vi "InstrumentControl.vi"(1 "Close VISA?":bool, 3 "Position":refnum<vi>, 5 "Status":refnum<vi>, 6 "Home fail":refnum<vi>, 7 "Busy":refnum<vi>, 8 "error":errorcluster, 9 "Open VISA?":bool, 10 "Input Message":string, 11 "HomeDone":refnum<vi>) -> (0 "error out":errorcluster, 2 "Output Message":string)   [LabVIEW 2018]
uses:
  QuickSilver/QuickSilver.lvclass
  D:/AOPD/TCSPD/Versoes TCSPD/21 - 160 - TCSPD_TRABALHO_BACKUP 2025-05-19/TCSPD_TRABALHO/Coude/Device/Device.lvclass
  Controlador/Motor/Motor.lvclass
  Controlador/Rele/Rele.lvclass
  Device/Device.lvclass
  Controlador/Comm/COMM.lvclass
  <vilib>/Utility/error.llb/DialogType.ctl
panel:
  in  "UART1":refnum<class "COMM.lvclass">
  in  "Device.lvclass":refnum<class "Device.lvclass">
  in  "LAMPADA":refnum<class "Rele.lvclass">
  in  "REDE":refnum<class "Motor.lvclass">
  in  "ESPELHO":refnum<class "QuickSilver.lvclass">
  in  "PRISMA":refnum<class "QuickSilver.lvclass">
  in  "FENDA":refnum<class "QuickSilver.lvclass">
  out "PAR":string
  out "CMD":string
  out "MEC":string
  # "Objects from Device -> Controlador class"
  # "Objects from Device -> QuickSilver class"
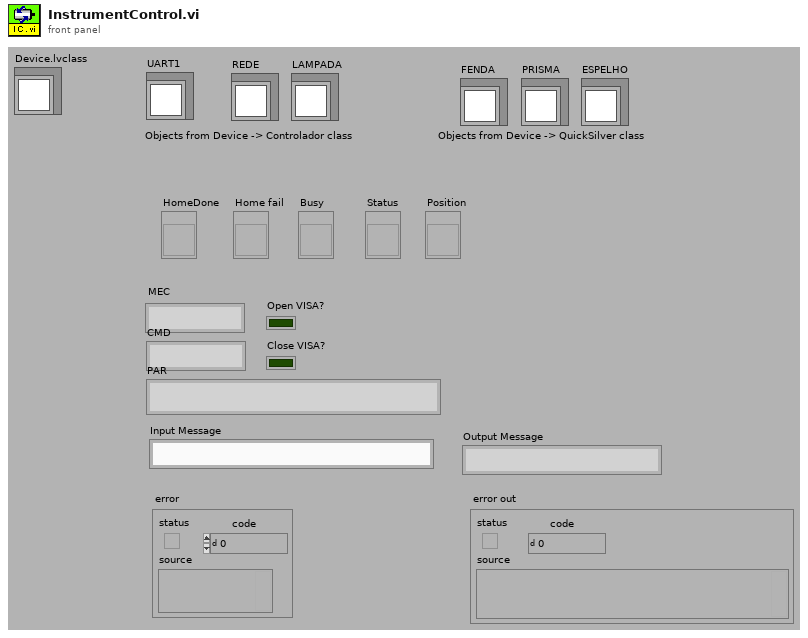
[diagram p1: front panel]
types:
  T1 = typedef "DialogType.ctl" = u16
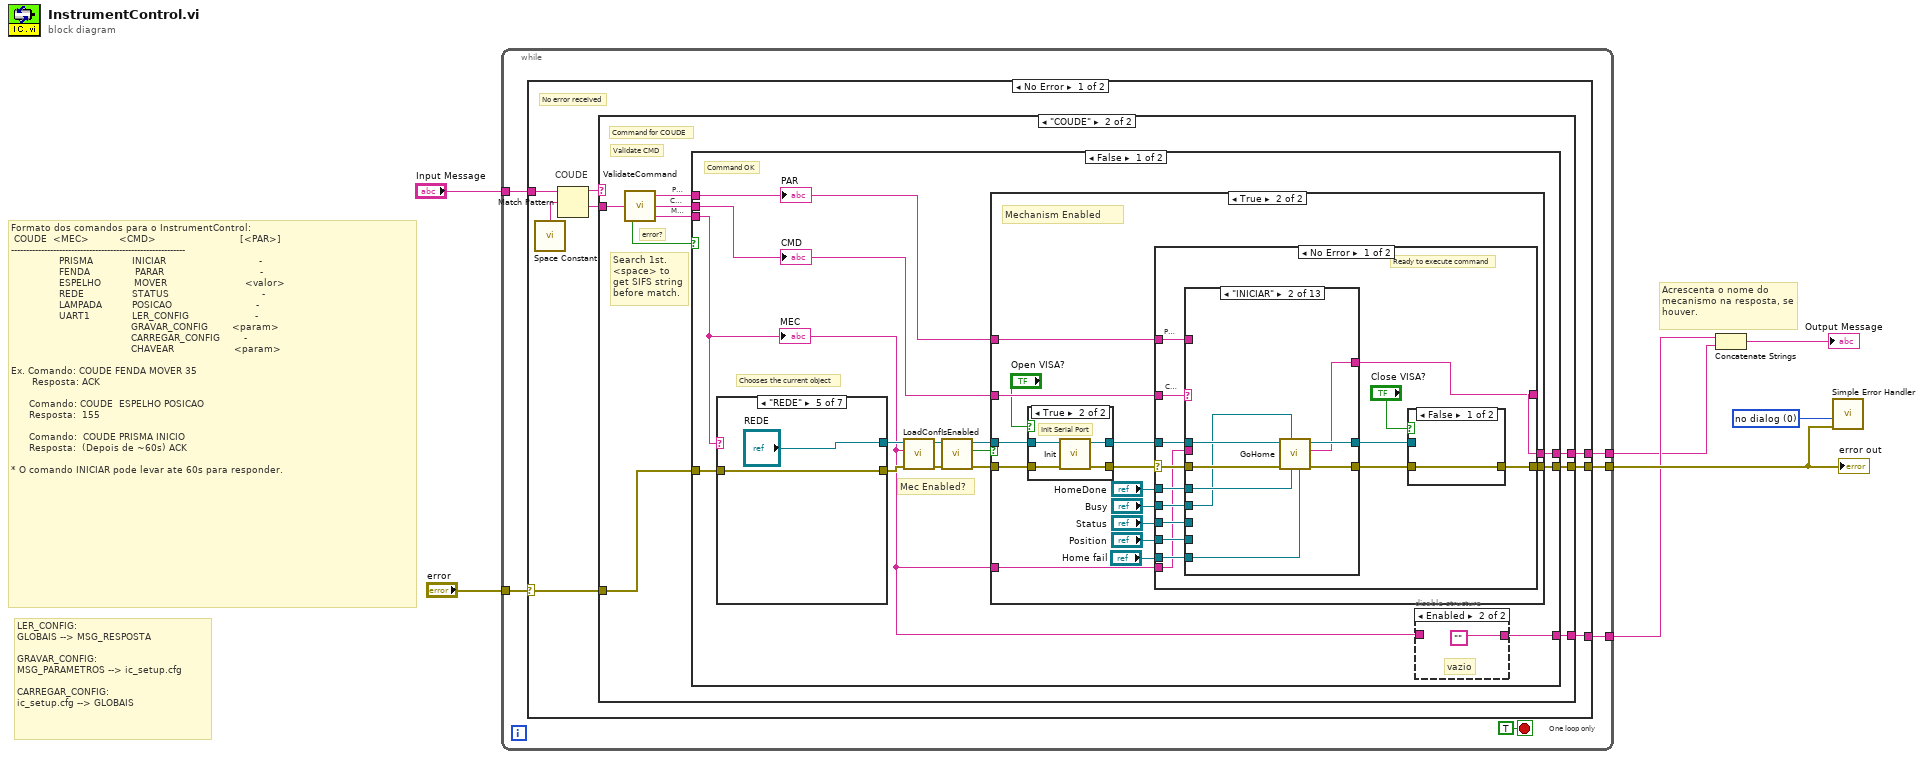
[diagram p0: block diagram]
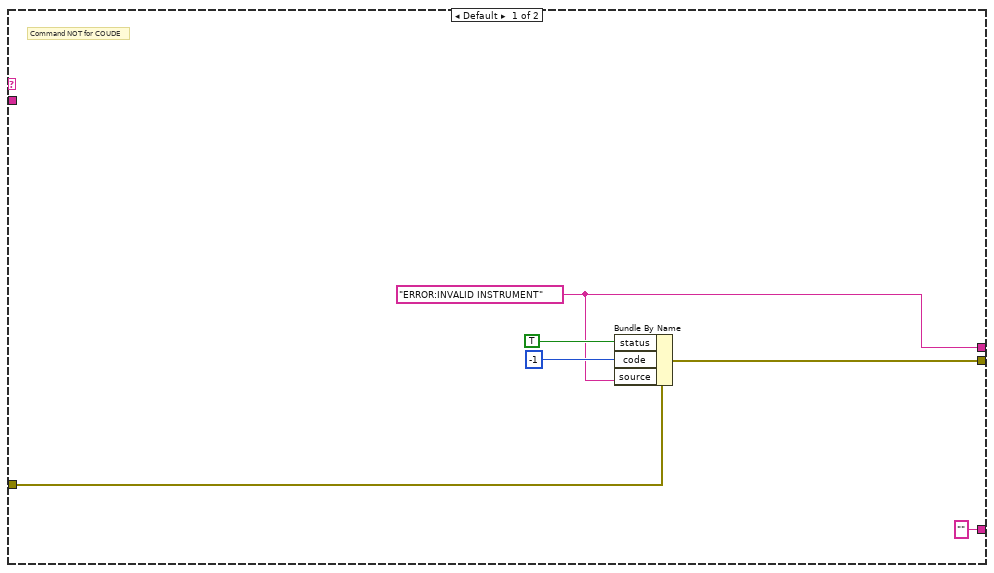
[diagram p2: hidden frame]
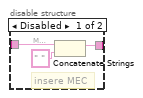
[diagram p3: hidden frame]
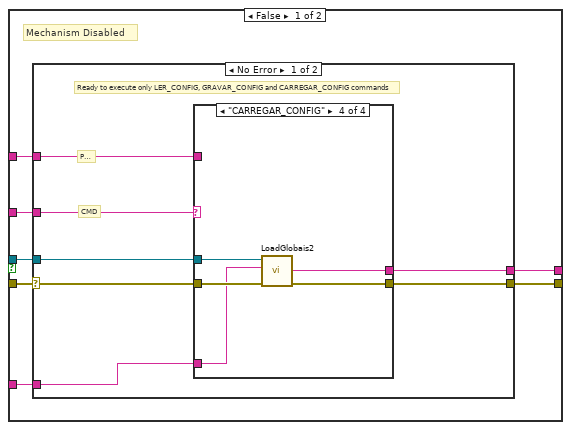
[diagram p4: hidden frame]
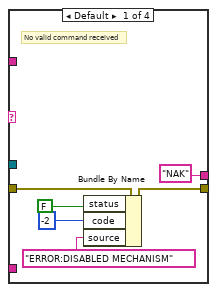
[diagram p5: hidden frame]
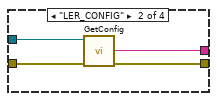
[diagram p6: hidden frame]
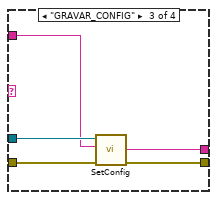
[diagram p7: hidden frame]
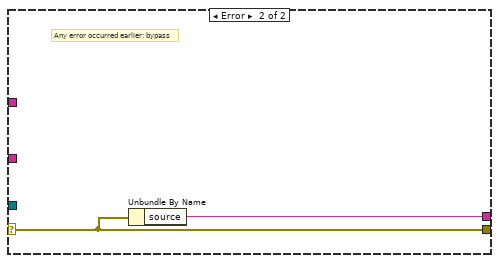
[diagram p8: hidden frame]
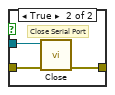
[diagram p10: hidden frame]
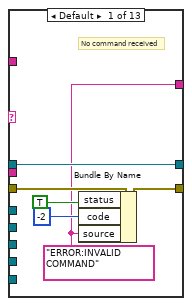
[diagram p11: hidden frame]
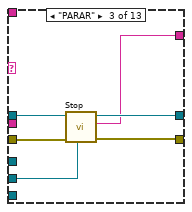
[diagram p12: hidden frame]
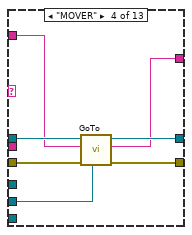
[diagram p13: hidden frame]
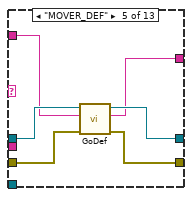
[diagram p14: hidden frame]
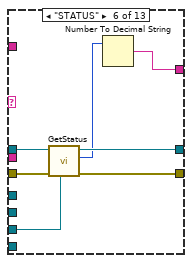
[diagram p15: hidden frame]
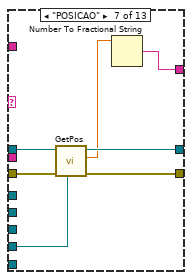
[diagram p16: hidden frame]
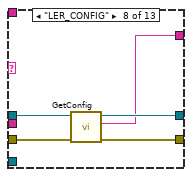
[diagram p17: hidden frame]
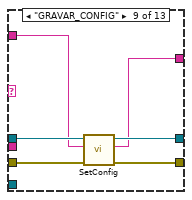
[diagram p18: hidden frame]
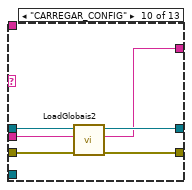
[diagram p19: hidden frame]
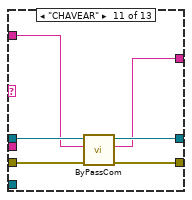
[diagram p20: hidden frame]
diagram:
  w7 = T1 0 items=["no dialog", "OK message", "continue or stop message", "OK message + warnings", "continue/stop + warnings"] ("type of dialog (OK msg:1)")
  # "LER_CONFIG:\nGLOBAIS --> MSG_RESPOSTA\n\nGRAVAR_CONFIG:\nMSG_PARAMETROS --> ic_setup.cfg\n\nCARREGAR_CONFIG:\nic_setup.cfg --> GLOBAIS"
  # "Acrescenta o nome do mecanismo na resposta, se houver."
  # "Formato dos comandos para o InstrumentControl:\n COUDE  <MEC>          <CMD>                            [<PAR>]\n----------------------------------------------------------\n                PRISMA             INICIAR                               -\n                FENDA               PARAR                                -  \n                ESPELHO           MOVER                          <valor>                 \n                REDE                STATUS                               -\n                LAMPADA          POSICAO                            -\n                UART1              LER_CONFIG                      -\n                                        GRAVAR_CONFIG        <param>\n                                        CARREGAR_CONFIG        -\n                                        CHAVEAR                    <param>\n          \nEx. Comando: COUDE FENDA MOVER 35\n       Resposta: ACK\n    \n      Comando: COUDE  ESPELHO POSICAO\n      Resposta:  155\n\n      Comando:  COUDE PRISMA INICIO\n      Resposta:  (Depois de ~60s) ACK \n\n* O comando INICIAR pode levar ate 60s para responder."
  n1 = while {
    tunnel: [w10] -> w6
    tunnel: "Input Message" -> [w12]
    tunnel: "error" -> [w11]
    tunnel: [w9] -> w3
    tunnel: [w8] -> w1
    stop <- TRUE ("stop") stop-if-true
    # "One loop only"
    n2 = case shown="No Error" w11 {
      selector: w11 -> [w21 w239]
      tunnel: [w17 w239] -> w10
      tunnel: w12 -> [w16 _]
      tunnel: [w15 ""] -> w9
      tunnel: [w14 "NAK"] -> w8
      frame No Error {
        # "No error received"
        # "COUDE"
        n3 = call <vilib>:"Space Constant.vi"() -> ("String"=w20:string)
        n4 = Match Pattern(string=w16, regular expression=w20) -> (before substring=w18:string, after substring=w19:string)  [unwired: 3 out]
        n5 = case shown="\"COUDE\"" w18 {
          tunnel: w19 -> [_ w36]
          tunnel: w21 -> [w24 w31]
          tunnel: [w25 w30] -> w17
          tunnel: ["" w29] -> w15
          tunnel: [w22 w28] -> w14
          frame Default {
            w22 = "ERROR:INVALID INSTRUMENT" ("source")
            # "Command NOT for COUDE"
            n6 = Bundle By Name(cluster=w24, "status"=TRUE, "code"=-1, "source"=w22) -> (w25:errorcluster)
          }
          frame "COUDE" {
            # "Search 1st.\n<space> to\nget SIFS string\nbefore match."
            # "MEC"
            # "CMD"
            # "PAR"
            # "Command for COUDE"
            # "Validate CMD"
            # "error?"
            n7 = call "ValidateCommand.vi"("input message 4"=w36) -> ("MECH"=w32:string, "CMD"=w33:string, "PARAM"=w34:string, "err_out"=w35:bool)  [unwired: 1 out]
            n8 = case shown="False" w35 {
              tunnel: w34 -> [w50 _]
              tunnel: w33 -> [w49 _]
              tunnel: w32 -> [w37 _]
              tunnel: w31 -> [w48 w236]
              tunnel: [w45 w235] -> w30
              tunnel: [w39 ""] -> w29
              tunnel: [w38 w231] -> w28
              frame False {
                # "Mec Enabled?"
                # "Chooses the current object"
                # "Command OK"
                n9 = case shown="\"REDE\"" w37 {
                  tunnel: w48 -> [w215 w220 w221 w223 w226 w227 w230]
                  tunnel: [w214 w220 w221 w223 w226 w227 w230] -> w46
                  tunnel: ["Device.lvclass" "FENDA" "PRISMA" "ESPELHO" "REDE" "LAMPADA" "UART1"] -> w47
                  frame Default {
                    # "No valid mechanism received"
                    n10 = Bundle By Name(cluster=w215, "status"=TRUE, "code"=-1, "source"="NAK : INVALID MECHANISM") -> (w214:errorcluster)
                  }
                  frame "FENDA" {
                  }
                  frame "PRISMA" {
                  }
                  frame "ESPELHO" {
                  }
                  frame "REDE" {
                  }
                  frame "LAMPADA" {
                  }
                  frame "SERIAL" {
                  }
                }
                n11 = call-dynamic "LoadConf.vi"("error in"=w46, "MEC"=w37, "Device in"=w47) -> ("error out"=w43:errorcluster, "Device out"=w44:refnum<class "Device.lvclass">)  [unwired: 7 out]
                n12 = call-dynamic "IsEnabled.vi"("error in (no error)"=w43, "Device in"=w44) -> ("error out"=w40:errorcluster, "Boolean"=w42:bool, "Device out"=w41:refnum<class "Device.lvclass">)  [unwired: 7 out]
                n13 = case shown="True" w42 {
                  tunnel: w50 -> [w61 w104]
                  tunnel: w49 -> [w60 w103]
                  tunnel: [w57 w102] -> w45
                  tunnel: w41 -> [w59 w96]
                  tunnel: w40 -> [w58 w94]
                  tunnel: [w56 w92] -> w38
                  tunnel: w37 -> [w55 w91]
                  frame False {
                    # "Mechanism Disabled"
                    n14 = case shown="No Error" w58 {
                      selector: w58 -> [w66 w90]
                      tunnel: w60 -> [w65 _]
                      tunnel: w61 -> [w68 _]
                      tunnel: w59 -> [w67 _]
                      tunnel: [w64 w90] -> w57
                      tunnel: [w63 w89] -> w56
                      tunnel: w55 -> [w62 _]
                      frame No Error {
                        # "Ready to execute only LER_CONFIG, GRAVAR_CONFIG and CARREGAR_CONFIG commands"
                        # "PAR"
                        # "CMD"
                        n15 = case shown="\"CARREGAR_CONFIG\"" w65 {
                          tunnel: w68 -> [_ _ w81 _]
                          tunnel: w67 -> [_ w78 w83 w88]
                          tunnel: w66 -> [w72 w77 w82 w86]
                          tunnel: [w71 w76 w80 w85] -> w64
                          tunnel: ["NAK" ("Resp") w75 w79 w87] -> w63
                          tunnel: w62 -> [_ _ _ w84]
                          frame Default {
                            # "No valid command received"
                            n16 = Bundle By Name(cluster=w72, "status"=FALSE, "code"=-2, "source"="ERROR:DISABLED MECHANISM") -> (w71:errorcluster)
                          }
                          frame "LER_CONFIG" {
                            n17 = call-dynamic "GetConfig.vi"("error in (no error)"=w77, "Device in"=w78) -> ("error out"=w76:errorcluster, "Resp"=w75:string)  [unwired: 7 in, 1 out]
                          }
                          frame "GRAVAR_CONFIG" {
                            n18 = call-dynamic "SetConfig.vi"("error in (no error)"=w82, "PARAM"=w81, "Device in"=w83) -> ("error out"=w80:errorcluster, "RESP"=w79:string)  [unwired: 7 out]
                          }
                          frame "CARREGAR_CONFIG" {
                            n19 = call-dynamic "LoadGlobais2.vi"("error in (no error)"=w86, "Mecanismo"=w84, "Device in"=w88) -> ("error out"=w85:errorcluster, "Resp"=w87:string)  [unwired: 6 in, 1 out]
                          }
                        }
                      }
                      frame Error {
                        # "Any error occurred earlier: bypass"
                        n20 = Unbundle By Name(w90) -> ("source"=w89:string)
                      }
                    }
                  }
                  frame True {
                    # "Mechanism Enabled"
                    n21 = case shown="True" "Open VISA?" {
                      tunnel: [w107 w111] -> w105
                      tunnel: w96 -> [w107 w110]
                      tunnel: w94 -> [w106 w109]
                      tunnel: [w106 w108] -> w93
                      frame False {
                      }
                      frame True {
                        # "Init Serial Port"
                        n22 = call-dynamic "Init.vi"("error in (no error)"=w109, "Device in"=w110) -> ("error out"=w108:errorcluster, "Device out"=w111:refnum<class "Device.lvclass">)  [unwired: 8 out]
                      }
                    }
                    n23 = case shown="No Error" w93 {
                      selector: w93 -> [w124 w212]
                      tunnel: w103 -> [w120 _]
                      tunnel: w104 -> [w126 _]
                      tunnel: w105 -> [w125 _]
                      tunnel: [w123 w212] -> w102
                      tunnel: [w113 w211] -> w92
                      tunnel: "Status" -> [w119 _]
                      tunnel: "HomeDone" -> [w118 _]
                      tunnel: "Busy" -> [w117 _]
                      tunnel: "Position" -> [w116 _]
                      tunnel: "Home fail" -> [w115 _]
                      tunnel: w91 -> [w112 _]
                      frame No Error {
                        # "Ready to execute command"
                        # "PAR"
                        # "CMD"
                        n24 = case shown="\"INICIAR\"" w120 {
                          tunnel: w126 -> [_ _ _ w153 w162 _ _ _ w186 _ w195 _ _]
                          tunnel: w125 -> [w132 w144 w150 w157 w163 w170 w177 w182 w188 w194 w200 w205 w210]
                          tunnel: w124 -> [w134 w143 w149 w156 w161 w169 w176 w181 w187 w193 w199 w202 w209]
                          tunnel: [w132 w141 w148 w154 w159 w167 w175 w180 w185 w192 w198 w203 w207] -> w121
                          tunnel: [w133 w142 w147 w155 w160 w168 w174 w179 w184 w191 w197 w201 w208] -> w122
                          tunnel: [w131 w137 w145 w151 w158 w164 w171 w178 w183 w190 w196 w204 w206] -> w113
                          tunnel: w119 -> [_ _ _ _ _ w166 _ _ _ _ _ _ _]
                          tunnel: w118 -> [_ w140 _ _ _ _ _ _ _ _ _ _ _]
                          tunnel: w117 -> [_ w138 w146 w152 _ _ _ _ _ _ _ _ _]
                          tunnel: w116 -> [_ _ _ _ _ _ w172 _ _ _ _ _ _]
                          tunnel: w115 -> [_ w139 _ _ _ _ _ _ _ _ _ _ _]
                          tunnel: w112 -> [_ _ _ _ _ _ _ _ _ w189 _ _ _]
                          frame Default {
                            w131 = "ERROR:INVALID COMMAND" ("source")
                            # "No command received"
                            n25 = Bundle By Name(cluster=w134, "status"=TRUE, "code"=-2, "source"=w131) -> (w133:errorcluster)
                          }
                          frame "INICIAR" {
                            n26 = call-dynamic "GoHome.vi"("Home fail"=w139, "HomeDone"=w140, "Busy"=w138, "error in (no error)"=w143, "Device in"=w144) -> ("error out"=w142:errorcluster, "String"=w137:string, "Device out"=w141:refnum<class "Device.lvclass">)  [unwired: 4 out]
                          }
                          frame "PARAR" {
                            n27 = call-dynamic "Stop.vi"("Busy"=w146, "error in (no error)"=w149, "Device in"=w150) -> ("error out"=w147:errorcluster, "String"=w145:string, "Device out"=w148:refnum<class "Device.lvclass">)  [unwired: 6 out]
                          }
                          frame "MOVER" {
                            n28 = call-dynamic "GoTo.vi"("Busy"=w152, "error in (no error)"=w156, "Param"=w153, "Device in"=w157) -> ("error out"=w155:errorcluster, "Response"=w151:string, "Device out"=w154:refnum<class "Device.lvclass">)  [unwired: 5 out]
                          }
                          frame "MOVER_DEF" {
                            n29 = call-dynamic "GoDef.vi"("error in (no error)"=w161, "String 2"=w162, "Device in"=w163) -> ("error out"=w160:errorcluster, "String"=w158:string, "Device out"=w159:refnum<class "Device.lvclass">)  [unwired: 6 in]
                          }
                          frame "STATUS" {
                            n30 = call-dynamic "GetStatus.vi"("Stat Bin"=w166, "error in (no error)"=w169, "Device in"=w170) -> ("error out"=w168:errorcluster, "Status Int"=w165:i32, "Device out"=w167:refnum<class "Device.lvclass">)  [unwired: 6 out]
                            n31 = Number To Decimal String(number=w165) -> (decimal integer string=w164:string)  [unwired: 1 out]
                          }
                          frame "POSICAO" {
                            n32 = call-dynamic "GetPos.vi"("Position 2"=w172, "error in (no error)"=w176, "Device in"=w177) -> ("error out"=w174:errorcluster, "Position"=w173:dbl, "Device out"=w175:refnum<class "Device.lvclass">)  [unwired: 6 out]
                            n33 = Number To Fractional String(number=w173) -> (F-format string=w171:string)  [unwired: 3 out]
                          }
                          frame "LER_CONFIG" {
                            n34 = call-dynamic "GetConfig.vi"("error in (no error)"=w181, "Device in"=w182) -> ("error out"=w179:errorcluster, "Resp"=w178:string, "Device out"=w180:refnum<class "Device.lvclass">)  [unwired: 7 in]
                          }
                          frame "GRAVAR_CONFIG" {
                            n35 = call-dynamic "SetConfig.vi"("error in (no error)"=w187, "PARAM"=w186, "Device in"=w188) -> ("error out"=w184:errorcluster, "RESP"=w183:string, "Device out"=w185:refnum<class "Device.lvclass">)  [unwired: 6 out]
                          }
                          frame "CARREGAR_CONFIG" {
                            n36 = call-dynamic "LoadGlobais2.vi"("error in (no error)"=w193, "Mecanismo"=w189, "Device in"=w194) -> ("error out"=w191:errorcluster, "Resp"=w190:string, "Device out"=w192:refnum<class "Device.lvclass">)  [unwired: 6 in]
                          }
                          frame "CHAVEAR" {
                            n37 = call-dynamic "ByPassCom.vi"("error in (no error)"=w199, "Param"=w195, "Device in"=w200) -> ("error out"=w197:errorcluster, "Resp"=w196:string, "Device out"=w198:refnum<class "Device.lvclass">)  [unwired: 6 in]
                          }
                          frame "JOGCW" {
                            n38 = call-dynamic "JogCw.vi"("error in (no error)"=w202, "Device in"=w205) -> ("error out"=w201:errorcluster, "Response"=w204:string, "Device out"=w203:refnum<class "Device.lvclass">)  [unwired: 7 in]
                          }
                          frame "JOGCCW" {
                            n39 = call-dynamic "JogCcw.vi"("error in (no error)"=w209, "Device in"=w210) -> ("error out"=w208:errorcluster, "Response"=w206:string, "Device out"=w207:refnum<class "Device.lvclass">)  [unwired: 7 in]
                          }
                        }
                        n40 = case shown="False" "Close VISA?" {
                          tunnel: [w127 w130] -> w123
                          tunnel: w122 -> [w127 w129]
                          tunnel: w121 -> [_ w128]
                          frame False {
                          }
                          frame True {
                            # "Close Serial Port"
                            n41 = call-dynamic "Close.vi"("error in (no error)"=w129, "Device in"=w128) -> ("error out"=w130:errorcluster)  [unwired: 9 out]
                          }
                        }
                      }
                      frame Error {
                        # "Any error occurred earlier: bypass"
                        n42 = Unbundle By Name(w212) -> ("source"=w211:string)
                      }
                    }
                  }
                }
                n43 = disable-structure shown="Enabled" {
                  disable-tunnel: w37 -> [w53 _]
                  disable-tunnel: [w51 ""] -> w39
                  frame Disabled {
                    # "insere MEC"
                    # "MEC"
                    n44 = Concatenate Strings(w53, " " ("string")) -> (w51:string)
                  }
                  frame Enabled {
                    # "vazio"
                  }
                }
                "MEC" <- w37
                "CMD" <- w49
                "PAR" <- w50
              }
              frame True {
                w231 = "ERROR:INVALID COMMAND" ("source")
                # "Command NOT OK"
                n45 = Bundle By Name(cluster=w236, "status"=TRUE, "code"=-1, "source"=w231) -> (w235:errorcluster)
              }
            }
          }
        }
      }
      frame Error {
        # "\"Error in\" received: bypass"
      }
    }
  }
  "error out" <- w6
  n46 = Concatenate Strings(w3, w1) -> (→"Output Message":string)
  n47 = call <vilib>:"Simple Error Handler.vi"("type of dialog (OK msg:1)"=w7, "error in (no error)"=w6) -> ()  [unwired: 8 out]
